vi "Camera Optics Diagnostics_RC.vi"(8 "error in (no error)":errorcluster, 10 "Light Camera Info":T1, 11 "Rack Controller in":refnum<class "Rack Controller.lvclass">) -> (0 "error out":errorcluster, 3 "Rack Controller out":refnum<class "Rack Controller.lvclass">)   [LabVIEW 2019, in "Rack Controller.lvclass"]
uses:
  Rack Controller.lvclass
  Common/Controls/Camera Optics Diagnostics.ctl
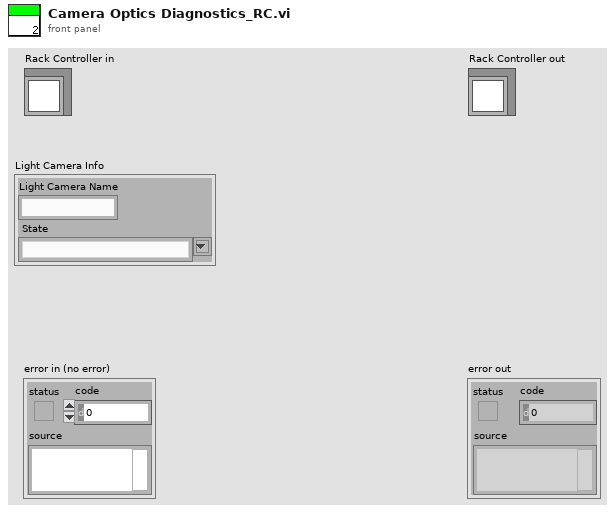
[diagram p1: front panel]
types:
  T1 = typedef "Camera Optics Diagnostics.ctl" = cluster{"Light Camera Name":string, " State":string}
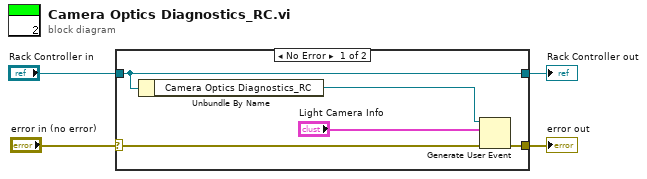
[diagram p0: block diagram]
diagram:
  n1 = case shown="No Error" "error in (no error)" {
    selector: "error in (no error)" -> [w6 w11]
    tunnel: [w5 w11] -> w3
    tunnel: [w9 w10] -> w1
    tunnel: "Rack Controller in" -> [w9 w10]
    frame No Error {
      n2 = Unbundle By Name(w9) -> ("Camera Optics Diagnostics_RC"=w8:refnum<user-event>)
      n3 = Generate User Event(user event=w8, event data cluster="Light Camera Info", error in=w6) -> (error out=w5:errorcluster)  [unwired: 1 in, 1 out]
    }
    frame Error {
    }
  }
  "error out" <- w3
  "Rack Controller out" <- w1
